vi "process scope.vi"(7 "data in":dbl[](array[numeric]), 8 "scope settings":T1, 9 "decimate":u16, 10 "Time Graph":refnum<vi>, 11 "Frequency Graph":refnum<vi>) -> ()   [LabVIEW 2018]
uses:
  scope settings.ctl
  <vilib>/Analysis/baseanly.llb/Mean (DBL).vi
  <vilib>/Analysis/4window.llb/Hanning Window (DBL).vi
  <vilib>/Analysis/2dsp.llb/Power Spectrum (DBL).vi
  <vilib>/Analysis/1siggen.llb/Ramp Pattern by Samples.vi
  <vilib>/Analysis/4window.llb/AllCosWindow (DBL).vi
  <vilib>/Analysis/NI_AALBase.lvlib
  <vilib>/Analysis/NI_AALPro.lvlib
panel:
  out "fifo adc in":dbl[](array[numeric])
  in  "store ratio":i16=4
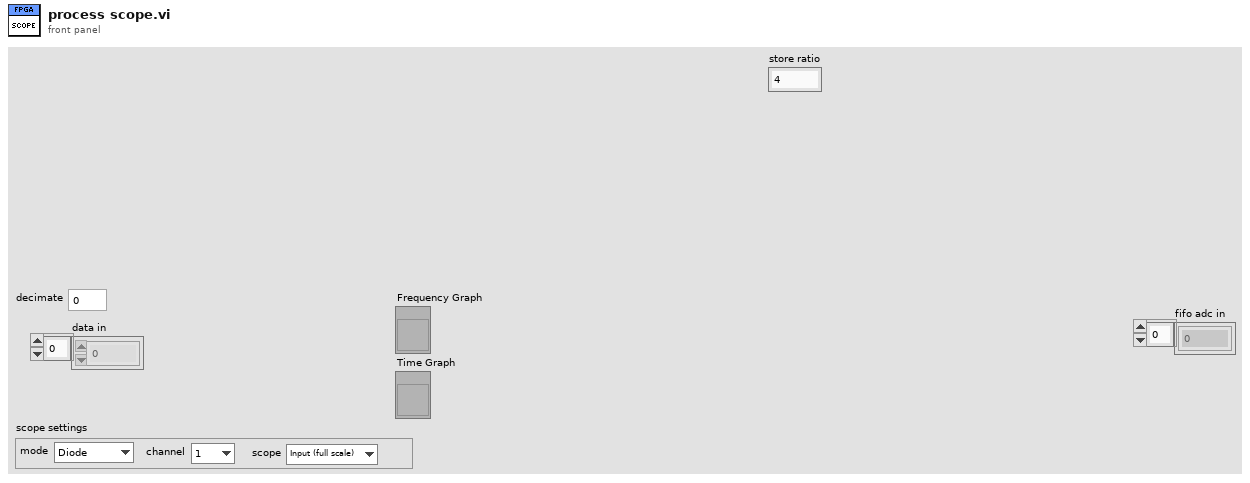
[diagram p1: front panel]
types:
  T1 = typedef "scope settings.ctl" = cluster{"mode":enum16{"Diode", "RF mixer", "lockin"}, "channel":enum16{"1", "2", "3"}, "scope":enum16{"Input (full scale)", "PLL out", "Phase error (deg)", "Freq. error (Hz)"}}
  T2 = enum16{"Input (full scale)", "PLL out", "Phase error (deg)", "Freq. error (Hz)"}
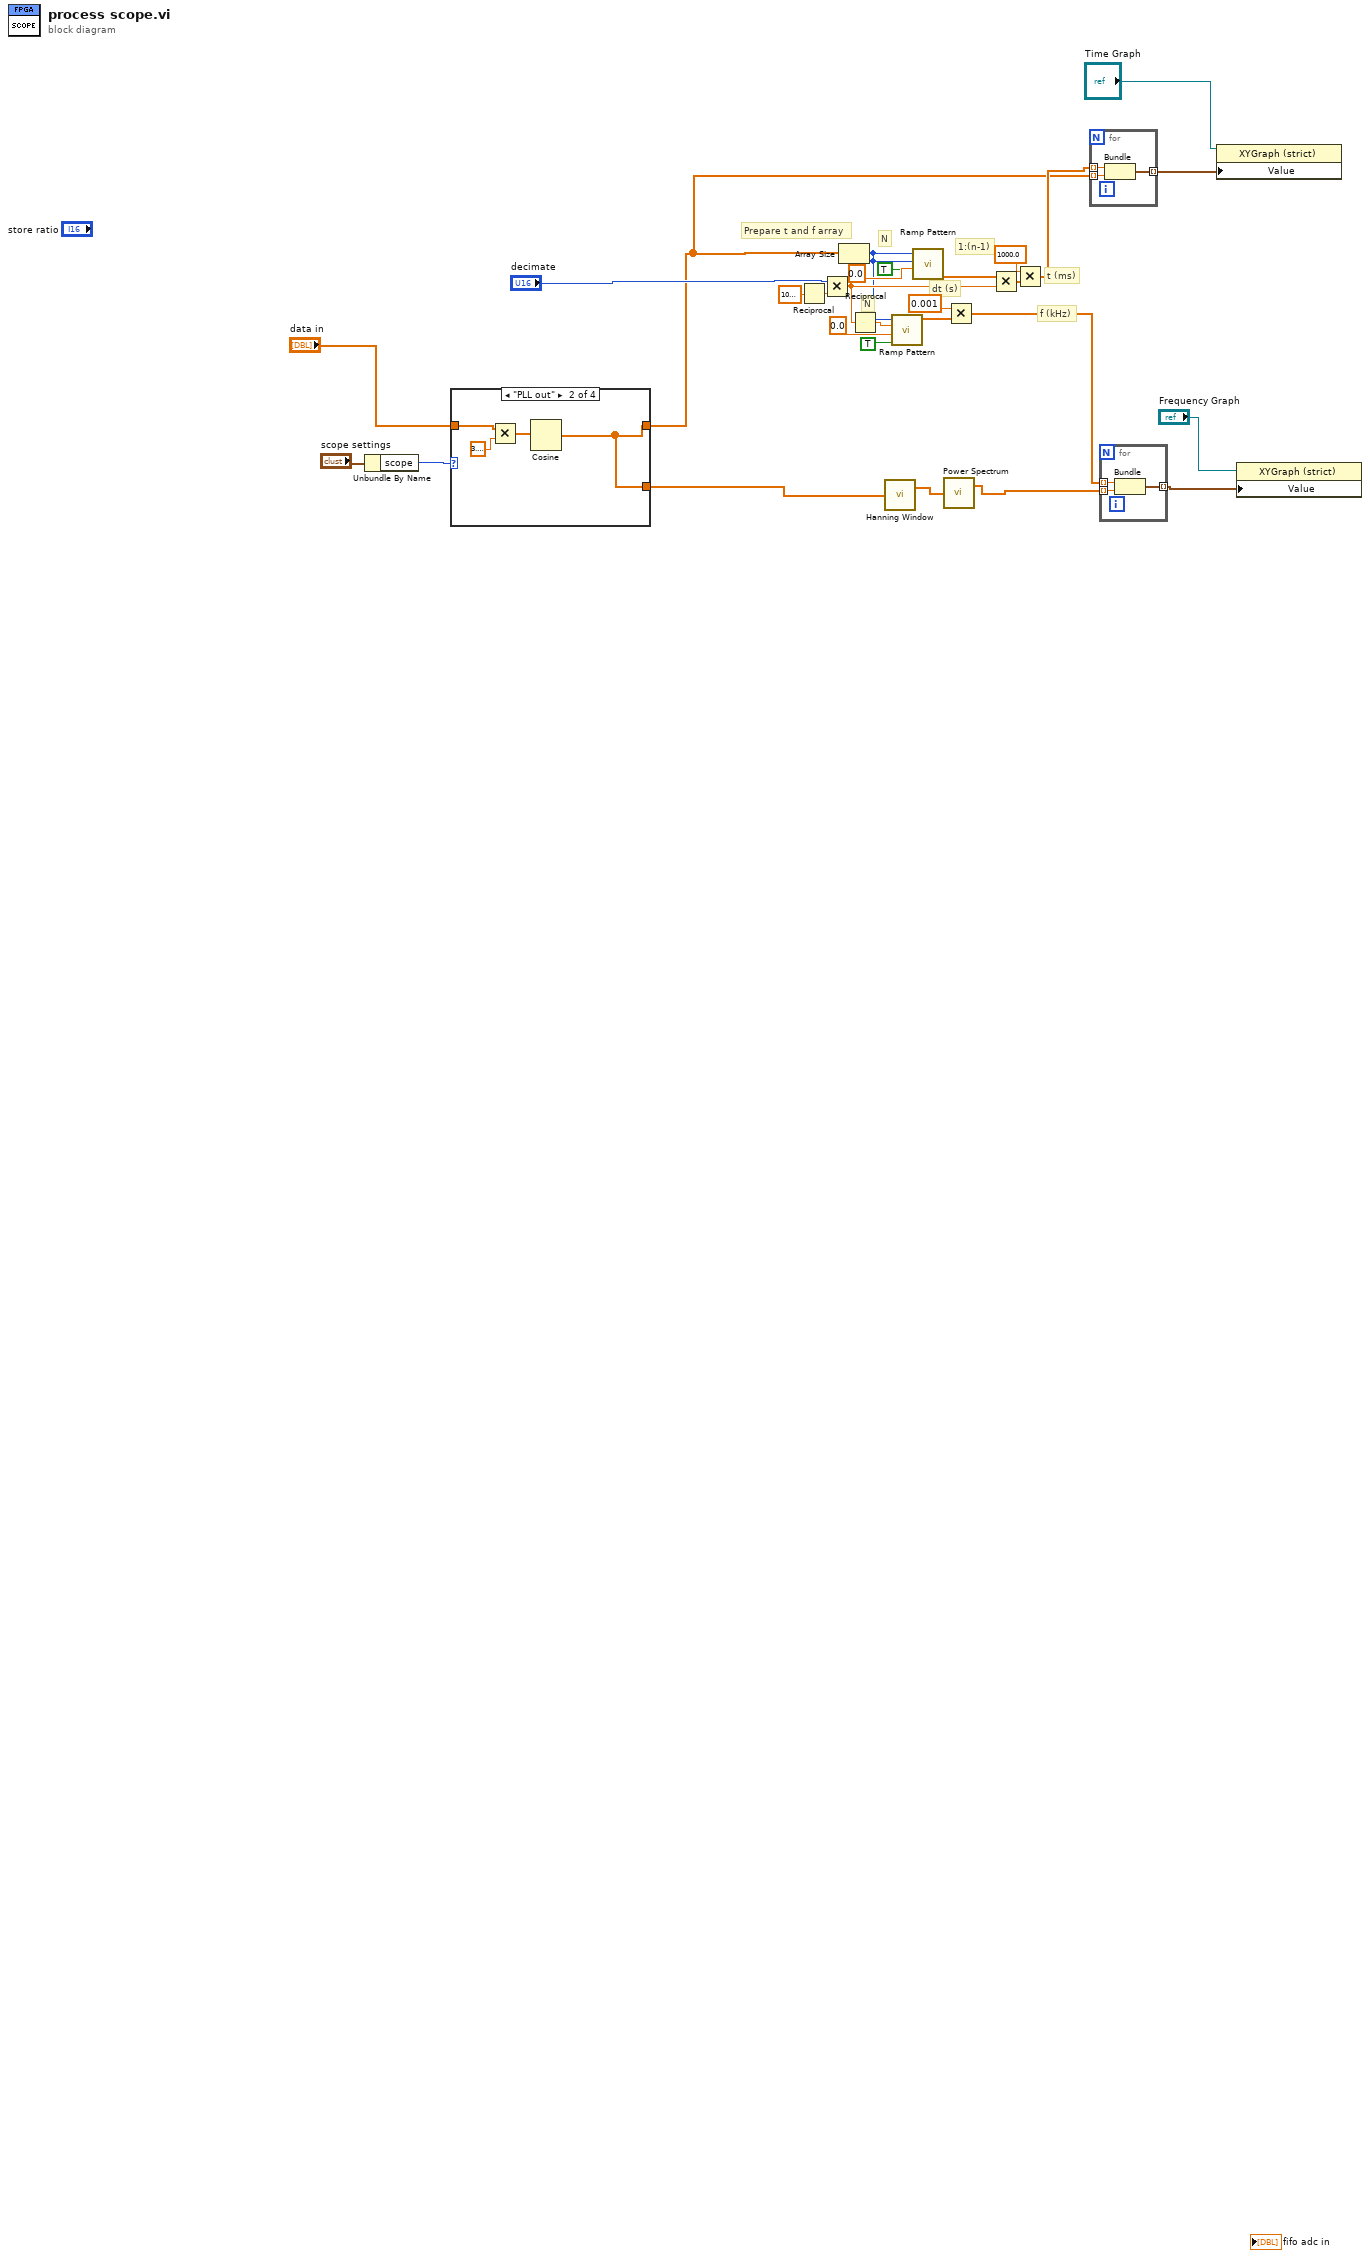
[diagram p0: block diagram]
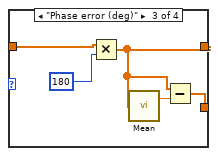
[diagram p3: hidden frame]
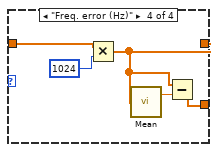
[diagram p4: hidden frame]
diagram:
  # "f (kHz)"
  # "t (ms)"
  # "Prepare t and f array"
  # "N"
  # "N"
  # "dt (s)"
  # "1:(n-1)"
  n1 = Unbundle By Name("scope settings") -> ("scope"=w7:T2)
  n2 = case shown="\"PLL out\"" w7 {
    tunnel: "data in" -> [w29 w33 w38 w43]
    tunnel: [w29 w30 w35 w40] -> w3
    tunnel: [w29 w30 w34 w39] -> w5
    frame "Input (full scale)", Default {
    }
    frame "PLL out" {
      n3 = Multiply(x=w33, y=3.141592653589793) -> (x*y=w31:dbl[])
      n4 = Cosine(x=w31) -> (cos(x)=w30:dbl[])
    }
    frame "Phase error (deg)" {
      n5 = Multiply(x=w38, y=180) -> (x*y=w35:dbl[])
      n6 = call-poly <vilib>:"Mean.vi"("X"=w35) -> ("mean"=w36:dbl)  [unwired: 1 out]
      n7 = Subtract(x=w35, y=w36) -> (x-y=w34:dbl[])
    }
    frame "Freq. error (Hz)" {
      n8 = Multiply(x=w43, y=1024) -> (x*y=w40:dbl[])
      n9 = call-poly <vilib>:"Mean.vi"("X"=w40) -> ("mean"=w41:dbl)  [unwired: 1 out]
      n10 = Subtract(x=w40, y=w41) -> (x-y=w39:dbl[])
    }
  }
  n11 = Reciprocal(x=1000000.0) -> (1/x=w28:dbl)
  n12 = Multiply(x="decimate", y=w28) -> (x*y=w19:dbl)
  n13 = Array Size(array=w3) -> (size(s)=w17:i32)
  n14 = Reciprocal(x=w19) -> (1/x=w18:dbl)
  n15 = call-poly <vilib>:"Hanning Window.vi"("X"=w5) -> ("Windowed X"=w14:dbl[])  [unwired: 1 out]
  n16 = call-poly <vilib>:"Ramp Pattern.vi"("exclude end?"=TRUE, "start"=0.0, "end"=w18, "samples"=w17) -> ("Ramp Pattern"=w16:dbl[])  [unwired: 6 in, 1 out]
  n17 = call-poly <vilib>:"Ramp Pattern.vi"("exclude end?"=TRUE, "start"=0.0, "end"=w17, "samples"=w17) -> ("Ramp Pattern"=w22:dbl[])  [unwired: 6 in, 1 out]
  n18 = call-poly <vilib>:"Power Spectrum.vi"("X"=w14) -> ("Power Spectrum"=w12:dbl[])  [unwired: 1 out]
  n19 = Multiply(x=0.001 ("start"), y=w16) -> (x*y=w13:dbl[])
  n20 = Multiply(x=w22, y=w19) -> (x*y=w23:dbl[])
  n21 = Multiply(x=1000.0, y=w23) -> (x*y=w4:dbl[])
  n22 = for {
    tunnel: w4 -> [w46] mode=indexing
    tunnel: w3 -> [w45] mode=indexing
    tunnel: [w44] -> w1 mode=indexing
    n23 = Bundle(w46, w45) -> (w44:cluster{dbl, dbl})  [unwired: 1 in]
  }
  n24 = for {
    tunnel: w13 -> [w49] mode=indexing
    tunnel: w12 -> [w48] mode=indexing
    tunnel: [w47] -> w9 mode=indexing
    n25 = Bundle(w49, w48) -> (w47:cluster{dbl, dbl})  [unwired: 1 in]
  }
  n26 = property class="XYGraph (strict)"(reference="Time Graph", "Value"=w1) -> ()  [unwired: 1 in, 2 out]
  n27 = property class="XYGraph (strict)"(reference="Frequency Graph", "Value"=w9) -> ()  [unwired: 1 in, 2 out]
